vi "GenerateTriggeredStimulus.vi"(8 "error in (no error)":errorcluster, 11 "Stimulus in":refnum<class "StimOnRailsThenOnTurns.lvclass">) -> (0 "error out":errorcluster, 2 "TriggeredStimulus":sgl[][](array[numeric]), 3 "Stimulus out":refnum<class "StimOnRailsThenOnTurns.lvclass">)   [LabVIEW 2019, in "StimOnRailsThenOnTurns.lvclass"]
uses:
  DetectSuppressionDuration/StimOnRailsThenOnTurns.lvclass
  WormTrackCluster.ctl
  StimulusObject.lvclass
  TrackTerminationReasonEnum.ctl
  DetectSuppressionDuration/StimOnRailsThenOnTurns.lvclass/StimOnRailsThenOnTurns.ctl
  ParametersGlobal.vi
panel:
  in  "Track":T1
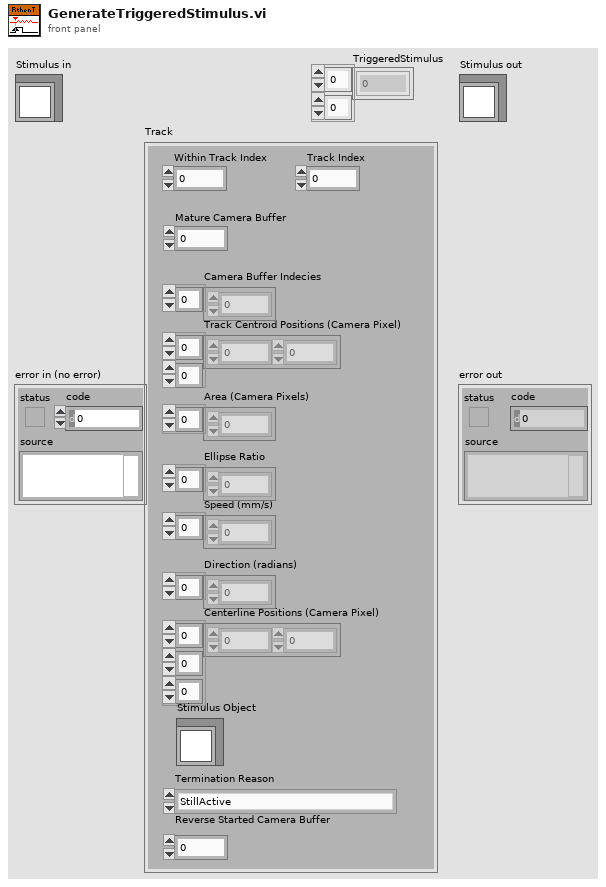
[diagram p1: front panel]
types:
  T1 = typedef "WormTrackCluster.ctl" = cluster{"Track Centroid Positions (Camera Pixel)":sgl[][], "Within Track Index":i32, "Camera Buffer Indecies":i32[], "Area (Camera Pixels)":i32[], "Speed (mm/s)":sgl[], "Direction (radians)":sgl[], "Centerline Positions (Camera Pixel)":sgl[][][], "Ellipse Ratio":sgl[], "Stimulus Object":refnum<class "StimulusObject.lvclass">, "Termination Reason":T2, "Track Index":i32, "Mature Camera Buffer":i32, "Reverse Started Camera Buffer":i32}
  T2 = typedef "TrackTerminationReasonEnum.ctl" = enum16{"StillActive", "MaxDisplacement", "NoBlobsLeft", "AreaIncrease", "AreaDecrease", "ExperimentEnded"}
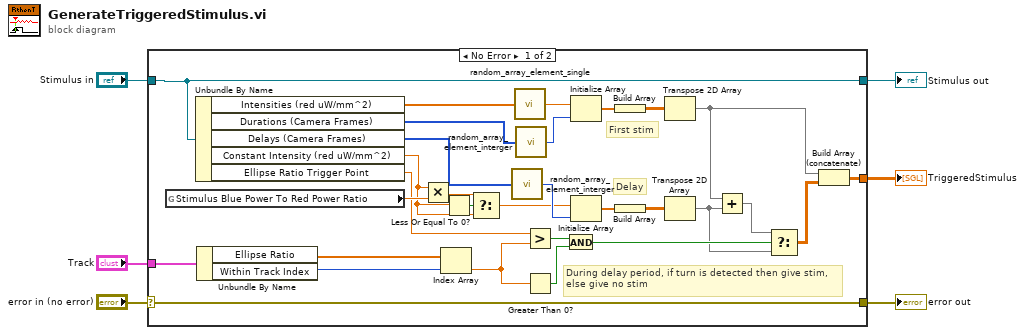
[diagram p0: block diagram]
diagram:
  n1 = case shown="No Error" "error in (no error)" {
    selector: "error in (no error)" -> [w36 w38]
    tunnel: [w36 w38] -> w2
    tunnel: [w20 w37] -> w4
    tunnel: "Stimulus in" -> [w20 w37]
    tunnel: [w8 _] -> w3
    tunnel: "Track" -> [w19 _]
    frame No Error {
      # "During delay period, if turn is detected then give stim, else give no stim"
      # "First stim"
      # "Delay"
      n2 = global read "ParametersGlobal.vi" "Stimulus Blue Power To Red Power Ratio"() -> (w24:sgl)
      n3 = Unbundle By Name(w20) -> ("Intensities (red uW/mm^2)"=w35:sgl[], "Durations (Camera Frames)"=w30:i32[], "Delays (Camera Frames)"=w21:i32[], "Constant Intensity (red uW/mm^2)"=w22:sgl, "Ellipse Ratio Trigger Point"=w15:sgl)
      n4 = Unbundle By Name(w19) -> ("Ellipse Ratio"=w14:sgl[], "Within Track Index"=w13:i32)
      n5 = Multiply(x=w22, y=w24) -> (x*y=w26:sgl)
      n6 = Index Array(array=w14, index=w13) -> (element=w16:sgl)
      n7 = Less Or Equal To 0?(x=w22) -> (x <= 0?=w25:bool)
      n8 = Select(t=w26, s=w25, f=w22) -> (s? t:f=w23:sgl)
      n9 = call "random_array_element_interger.vi"("Array of numbers"=w21) -> ("Randomly selected number"=w27:i32)
      n10 = call "random_array_element_single.vi"("Array of numbers"=w35) -> ("Randomly selected number"=w34:sgl)
      n11 = call "random_array_element_interger.vi"("Array of numbers"=w30) -> ("Randomly selected number"=w33:i32)
      n12 = Greater?(x=w15, y=w16) -> (0:w18:bool)
      n13 = Greater Than 0?(x=w16) -> (x > 0?=w17:bool)
      n14 = And(x=w18, y=w17) -> (x .and. y?=w12:bool)
      n15 = Initialize Array(w34, w33) -> (w32:sgl[])
      n16 = Initialize Array(w23, w27) -> (w29:sgl[])
      n17 = Build Array(w32) -> (w31:sgl[][])
      n18 = Build Array(w29) -> (w28:sgl[][])
      n19 = Transpose 2D Array(2D array=w31) -> (transposed array=w10:sgl[][])
      n20 = Transpose 2D Array(2D array=w28) -> (transposed array=w7:sgl[][])
      n21 = Add(x=w10, y=w7) -> (x+y=w11:sgl[][])
      n22 = Select(t=w11, s=w12, f=w7) -> (s? t:f=w9:sgl[][])
      n23 = Build Array (concatenate)(w10, w9) -> (w8:sgl[][])
    }
    frame Error {
    }
  }
  "error out" <- w2
  "Stimulus out" <- w4
  "TriggeredStimulus" <- w3
